vi "Create Folder at Location.vi"(5 "Override existing (F)":bool, 7 "Use Relative (F)":bool, 8 "Error In":errorcluster, 10 "Path":string) -> (0 "Error Out":errorcluster, 1 "Already Exists ?":bool, 2 "Full path out":path)   [LabVIEW 2019, in "gRPC Template Creation Utility.lvlib"]
uses:
  gRPC Template Creation Utility.lvlib
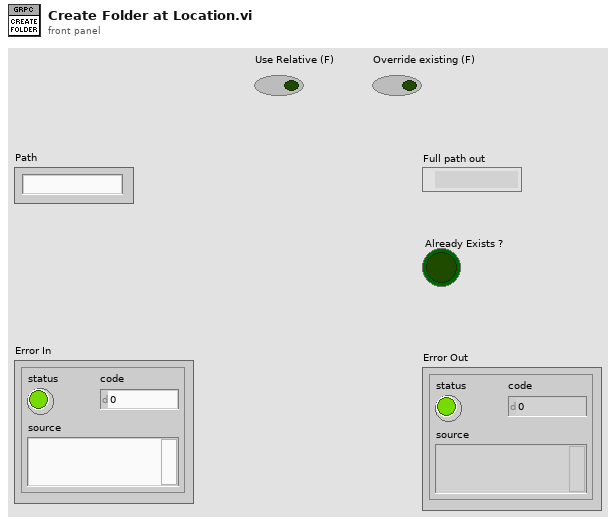
[diagram p1: front panel]
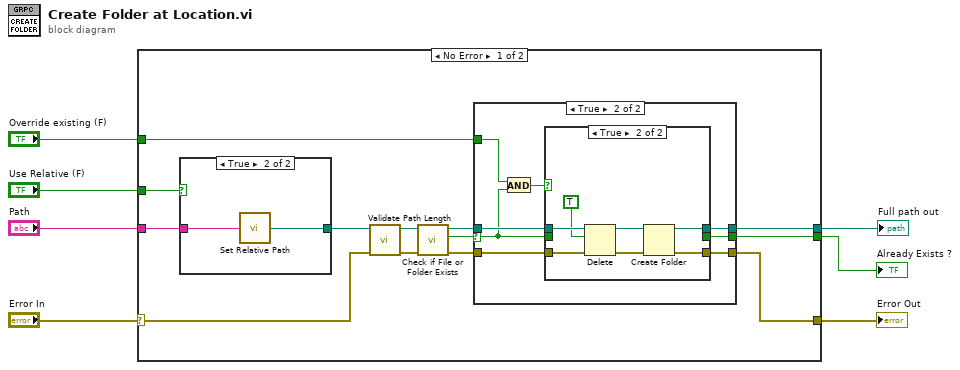
[diagram p0: block diagram]
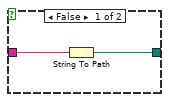
[diagram p2: hidden frame]
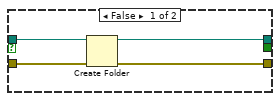
[diagram p3: hidden frame]
diagram:
  n1 = case shown="No Error" "Error In" {
    selector: "Error In" -> [w18 w47]
    tunnel: "Path" -> [w19 _]
    tunnel: "Use Relative (F)" -> [w20 _]
    tunnel: "Override existing (F)" -> [w14 _]
    tunnel: [w13 w47] -> w3
    tunnel: [w12 _] -> w2
    tunnel: [w11 _] -> w1
    frame No Error {
      n2 = case shown="True" w20 {
        tunnel: w19 -> [w22 w24]
        tunnel: [w21 w23] -> w9
        frame False {
          n3 = String To Path(string=w22) -> (path=w21:path)
        }
        frame True {
          n4 = call "Set Relative Path.vi"("Application Relative Path"=w24) -> ("Full Path"=w23:path)
        }
      }
      n5 = call "Validate Path Length.vi"("error in (no error)"=w18, "Path in"=w9) -> ("error out"=w10:errorcluster, "Path out"=w8:path)  [unwired: 8 in]
      n6 = call <vilib>:"Check if File or Folder Exists.vi"("error in (no error)"=w10, "path"=w8) -> ("error out"=w15:errorcluster, "file or folder exists?"=w17:bool, "dup path"=w16:path)  [unwired: 7 in]
      n7 = case shown="True" w17 {
        selector: w17 -> [_ w30]
        tunnel: w16 -> [w27 w36]
        tunnel: w15 -> [w28 w33]
        tunnel: w14 -> [_ w35]
        tunnel: [w25 w32] -> w12
        tunnel: [w26 w31] -> w13
        tunnel: [_ w29] -> w11
        frame False {
          n8 = Create Folder(path (use dialog)=w27, error in=w28) -> (created path=w25:path, error out=w26:errorcluster)  [unwired: 1 in, 1 out]
        }
        frame True {
          n9 = And(x=w35, y=w30) -> (x .and. y?=w34:bool)
          n10 = case shown="True" w34 {
            tunnel: w36 -> [w39 w46]
            tunnel: w33 -> [w38 w44]
            tunnel: [w38 w40] -> w31
            tunnel: [w39 w41] -> w32
            tunnel: w30 -> [w37 _]
            tunnel: [w37 _] -> w29
            frame False {
            }
            frame True {
              n11 = Delete(path (use dialog)=w46, entire hierarchy (F)=TRUE, error in=w44) -> (deleted path=w42:path, error out=w43:errorcluster)  [unwired: 2 in, 1 out]
              n12 = Create Folder(path (use dialog)=w42, error in=w43) -> (created path=w41:path, error out=w40:errorcluster)  [unwired: 1 in, 1 out]
            }
          }
        }
      }
    }
    frame Error {
    }
  }
  "Error Out" <- w3
  "Full path out" <- w2
  "Already Exists ?" <- w1
